vi "Encoder Counts to Degrees.vi"(9 "Post-Shaft Gear Ratio":dbl=1.0, 11 "Encoder Rotations":dbl) -> (3 "Degrees":dbl)   [LabVIEW 2015]
doc: "Converts count value from a (4096 count per rotation) encoder to degrees of a final output shaft."
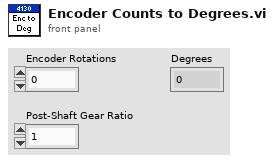
[diagram p1: front panel]
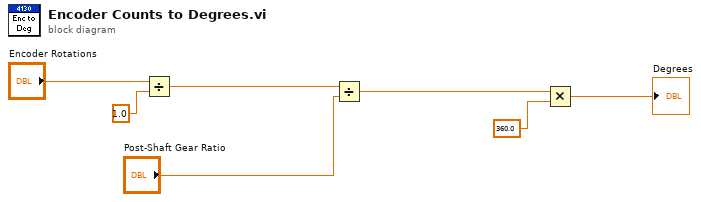
[diagram p0: block diagram]
diagram:
  n1 = Divide(x="Encoder Rotations", y=1.0 ("x")) -> (x/y=w3:dbl)
  n2 = Divide(x=w3, y="Post-Shaft Gear Ratio") -> (x/y=w6:dbl)
  n3 = Multiply(x=w6, y=360.0) -> (x*y=→"Degrees":dbl)
